vi "Shutdown.vi"(8 "error in (no error)":errorcluster, 11 "Motor Controller in":refnum<class "Motor Controller.lvclass">) -> (0 "error out":errorcluster, 3 "Motor Controller out":refnum<class "Motor Controller.lvclass">)   [LabVIEW 2022 SP3, in "Motor Controller.lvclass"]
uses:
  Motor Controller.lvclass
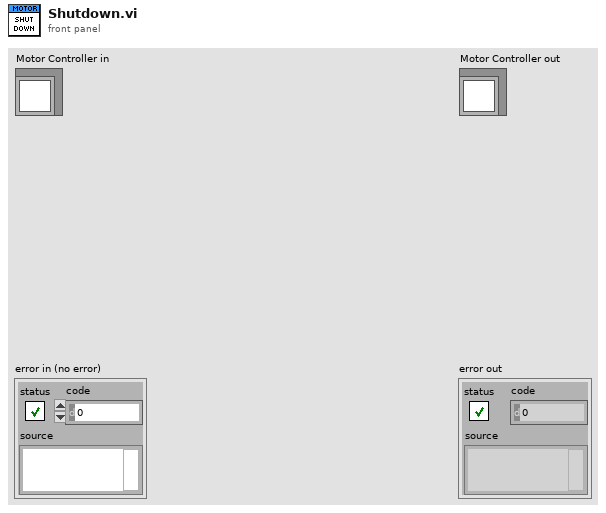
[diagram p1: front panel]
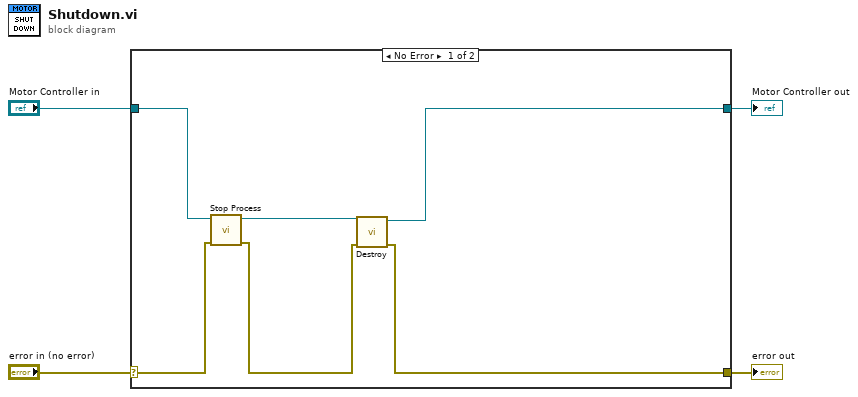
[diagram p0: block diagram]
diagram:
  n1 = case shown="No Error" "error in (no error)" {
    selector: "error in (no error)" -> [w10 w12]
    tunnel: [w5 w12] -> w3
    tunnel: [w8 w11] -> w1
    tunnel: "Motor Controller in" -> [w7 w11]
    frame No Error {
      n2 = call "Stop Process.vi"("error in (no error)"=w10, "Motor Controller in"=w7) -> ("error out"=w6:errorcluster, "Motor Controller out"=w9:refnum<class "Motor Controller.lvclass">)  [unwired: 8 in]
      n3 = call-dynamic "Destroy.vi"("error in (no error)"=w6, "Motor Controller in"=w9) -> ("error out"=w5:errorcluster, "Motor Controller out"=w8:refnum<class "Motor Controller.lvclass">)  [unwired: 8 in]
    }
    frame Error {
    }
  }
  "error out" <- w3
  "Motor Controller out" <- w1
